vi "validate.vi"(8 "error in":errorcluster, 11 "configuration in":refnum<class "channel configuration.lvclass">) -> (0 "error out":errorcluster, 3 "configuration out":refnum<class "channel configuration.lvclass">)   [LabVIEW 2013, in "channel configuration.lvclass"]
doc: "Provides an interface for performing validation on a given configuration. Any children should define the behavior of this function to ensure that the configuration in memory can be used by the runtime class."
uses:
  channel configuration.lvclass
  Configuration Framework/serializable configuration/NISE_CEF_serializable configuration.lvclass
  channel configuration.lvclass/channel configuration.ctl
  Configuration Framework/NISE_CEF_TreeControl.lvlib
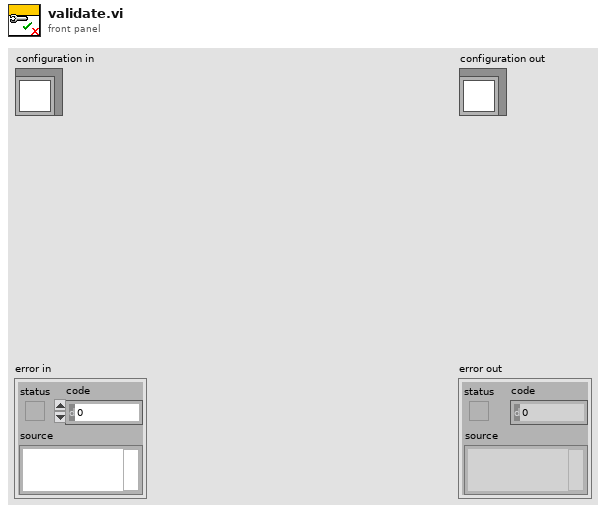
[diagram p1: front panel]
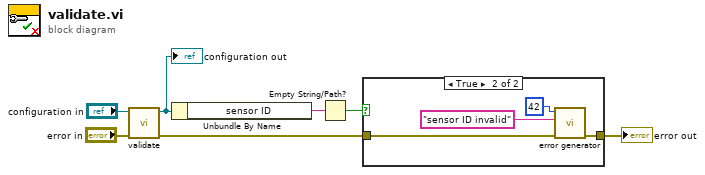
[diagram p0: block diagram]
diagram:
  n1 = call-parent "validate.vi"("error in"="error in", "configuration in"="configuration in") -> ("error out"=w2:errorcluster, "configuration out"=w5:refnum<class "channel configuration.lvclass">)  [unwired: 8 in]
  "configuration out" <- w5
  n2 = Unbundle By Name(w5) -> ("sensor ID"=w4:string)
  n3 = Empty String/Path?(string/path=w4) -> (empty?=w3:bool)
  n4 = case shown="True" w3 {
    tunnel: w2 -> [w8 w12]
    tunnel: [w8 w11] -> w1
    frame False {
    }
    frame True {
      n5 = call "error generator.vi"("error in"=w12, "append error message"="sensor ID invalid", "error code (0)"=42) -> ("error out"=w11:errorcluster)  [unwired: 6 in]
    }
  }
  "error out" <- w1
